vi "Equação de estado vão variavel.vi"(4 "A1 (m)":dbl=500.0, 5 "t2-t1 (°C)":dbl=35.0, 6 "To1 (N)":dbl=18350.0, 7 "Alfa t (1/°C)":dbl=2.09e-05, 8 "E (Pa)":dbl=65500000000.0, 9 "S (m²)":dbl=0.0005168, 10 "p (N/m)":dbl=18.35, 11 "Ao (m)":dbl=500.0) -> (2 "To2 Real  (N)":dbl=17749.49999999993 format="%.3f")   [LabVIEW 2020]
doc: "Calculo da tração com temperatura diferente da EDS"
panel:
  out "Numeric":i32
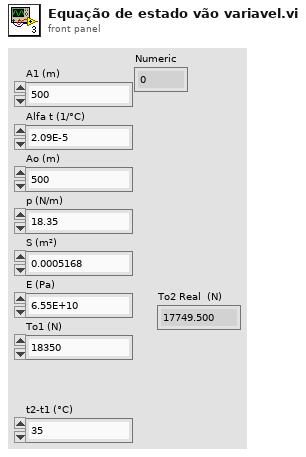
[diagram p1: front panel]
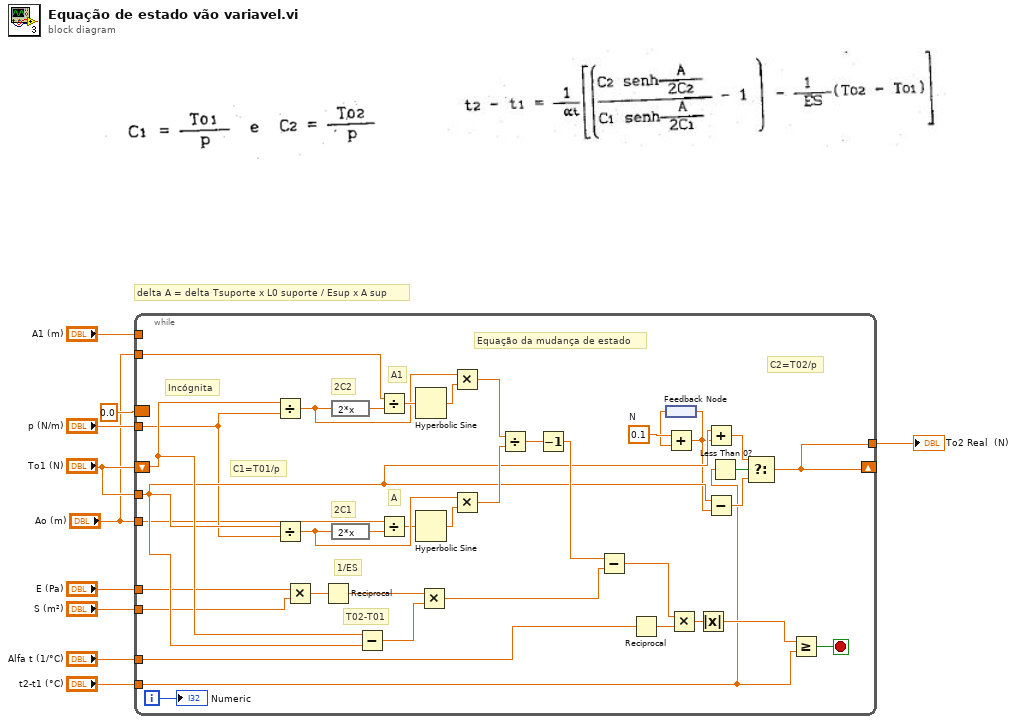
[diagram p0: block diagram]
diagram:
  # "delta A = delta Tsuporte x L0 suporte / Esup x A sup"
  n1 = while {
    shift-right: [w14] -> _
    shift-left: "To1 (N)" -> [w27]
    tunnel: "To1 (N)" -> [w22]
    border: 0.0 -> [_]
    tunnel: "E (Pa)" -> [w19]
    tunnel: "S (m²)" -> [w18]
    tunnel: "t2-t1 (°C)" -> [w17]
    tunnel: "Alfa t (1/°C)" -> [w16]
    tunnel: "p (N/m)" -> [w15]
    tunnel: [w14] -> w3
    tunnel: "Ao (m)" -> [w13]
    tunnel: "Ao (m)" -> [w12]
    tunnel: "A1 (m)" -> [_]
    i -> [w11]
    stop <- w26 stop-if-true
    w29 = 0.1  # N
    # "Equação da mudança de estado"
    # "Incógnita"
    # "T02-T01"
    # "1/ES"
    # "C1=T01/p"
    # "A"
    # "2C1"
    # "C2=T02/p"
    # "A1"
    # "2C2"
    n2 = Divide(x=w27, y=w15) -> (x/y=w45:dbl)
    n3 = Divide(x=w22, y=w15) -> (x/y=w44:dbl)
    n4 = Multiply(x=w19, y=w18) -> (x*y=w36:dbl)
    n5 = Reciprocal(x=w36) -> (1/x=w35:dbl)
    n6 = expression code="2*x"(w45) -> (w46:dbl)
    n7 = expression code="2*x"(w44) -> (w43:dbl)
    n8 = Subtract(x=w27, y=w22) -> (x-y=w34:dbl)
    n9 = Divide(x=w12, y=w46) -> (x/y=w48:dbl)
    n10 = Divide(x=w13, y=w43) -> (x/y=w41:dbl)
    n11 = Hyperbolic Sine(1:w48) -> (0:w47:dbl)
    n12 = Hyperbolic Sine(1:w41) -> (0:w42:dbl)
    n13 = Multiply(x=w35, y=w34) -> (x*y=w33:dbl)
    n14 = Multiply(x=w45, y=w47) -> (x*y=w40:dbl)
    n15 = Multiply(x=w44, y=w42) -> (x*y=w39:dbl)
    n16 = Divide(x=w40, y=w39) -> (x/y=w38:dbl)
    n17 = Decrement(x=w38) -> (x-1=w37:dbl)
    n18 = Subtract(x=w37, y=w33) -> (x-y=w32:dbl)
    n19 = Reciprocal(x=w16) -> (1/x=w31:dbl)
    n20 = feedback #1() -> (w28:dbl)
    n21 = Add(x=w29, y=w28) -> (x+y=w21:dbl)
    n22 = feedback-in #1(w21) -> ()
    n23 = Multiply(x=w32, y=w31) -> (x*y=w30:dbl)
    n24 = Absolute Value(x=w30) -> (abs(x)=w20:dbl)
    n25 = Add(x=w22, y=w21) -> (x+y=w23:dbl)
    n26 = Subtract(x=w22, y=w21) -> (x-y=w24:dbl)
    n27 = Less Than 0?(x=w17) -> (x < 0?=w25:bool)
    n28 = Select(t=w23, s=w25, f=w24) -> (s? t:f=w14:dbl)
    n29 = Greater Or Equal?(x=w20, y=w17) -> (x >= y?=w26:bool)
    "Numeric" <- w11
  }
  "To2 Real  (N)" <- w3
